vi "debugger Parse Query String.vi"(11 "ENV":T1) -> (1 "Serial Number":string, 2 "Model Number":string, 3 "Action":string)   [LabVIEW 2011]
uses:
  Addons/internet/utils/keyedarr.llb/Keyed Array.ctl
  Addons/internet/utils/strutil.llb/Case Matching.ctl
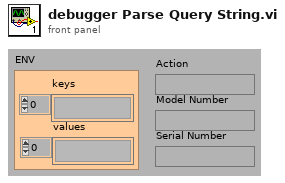
[diagram p1: front panel]
types:
  T1 = typedef "Keyed Array.ctl" = cluster{"keys":string[], "values":string[]}
  T2 = typedef "Case Matching.ctl" = enum16{"a != A", "a == A", "system"}
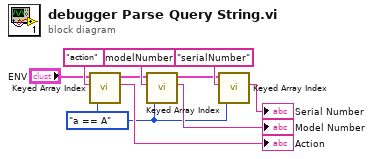
[diagram p0: block diagram]
diagram:
  w5 = Case_Matching."a == A" ("case matching (sensitive)")
  n1 = call "Keyed Array Index.vi"("case matching (sensitive)"=w5, "key"="action", "array in"="ENV") -> ("value"=→"Action":string, "duplicate array"=w2:T1)  [unwired: 1 in, 2 out]
  n2 = call "Keyed Array Index.vi"("case matching (sensitive)"=w5, "key"="modelNumber", "array in"=w2) -> ("value"=→"Model Number":string, "duplicate array"=w1:T1)  [unwired: 1 in, 2 out]
  n3 = call "Keyed Array Index.vi"("case matching (sensitive)"=w5, "key"="serialNumber", "array in"=w1) -> ("value"=→"Serial Number":string)  [unwired: 1 in, 3 out]
